vi "Run.vi"(8 "error in (no error)":errorcluster, 11 "SensorBase in":refnum<class "SensorBase.lvclass">) -> (0 "error out":errorcluster, 1 "DataValid":bool, 2 "clSensorData":T1, 3 "SensorBase out":refnum<class "SensorBase.lvclass">)   [LabVIEW 2018, in "SensorPlugins.lvlib" / "SensorBase.lvclass"]
uses:
  SensorBase.lvclass
  SensorShared/clSensorData.ctl
  <userlib>/NIST/BaseClasses/Object_class/BaseObject.lvclass
  SensorShared/SensorShared.lvlib
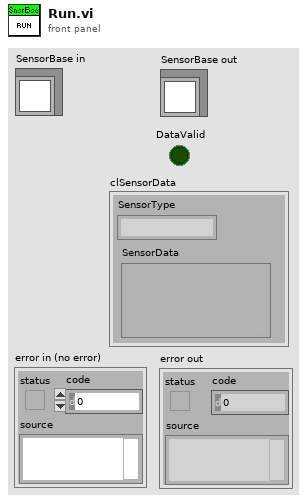
[diagram p1: front panel]
types:
  T1 = typedef "SensorShared.lvlib/clSensorData.ctl" = cluster{"SensorType":string, "SensorData":variant}
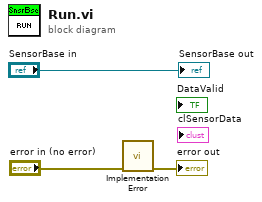
[diagram p0: block diagram]
diagram:
  n1 = call <userlib>:"Implementation Error.vi"("error in (no error)"="error in (no error)") -> ("error out"=→"error out":errorcluster)  [unwired: 10 in]
  "SensorBase out" <- "SensorBase in"
